vi "GT Buf Event Off.vi"(6 "fifo":i16, 7 "count":i16, 8 "error in (no error)":errorcluster caption="错误输入（无错误）", 9 "eventIndex":i16, 10 "crd":i16, 11 "cardNum":i16) -> (0 "error out":errorcluster caption="错误输出", 3 "function return":i16)   [LabVIEW 2020, in "gts1.lvlib"]
doc: "GT_API GT_BufEventOff(short cardNum,short crd,short eventIndex,short count,short fifo);"
uses:
  gts1.lvlib
  dll/32bit/multi_card/gts.dll
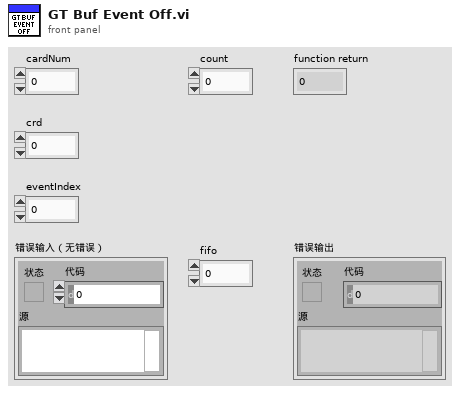
[diagram p1: front panel]
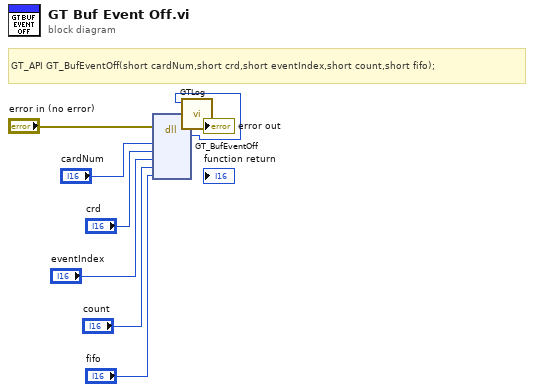
[diagram p0: block diagram]
diagram:
  # "GT_API GT_BufEventOff(short cardNum,short crd,short eventIndex,short count,short fifo);"
  n1 = dll-call lib="D:/Git/GoogolCard/dll/32bit/multi_card/gts.dll" fn="GT_BufEventOff"(error in="error in (no error)", "cardNum"="cardNum", "crd"="crd", "eventIndex"="eventIndex", "count"="count", "fifo"="fifo") -> (error out=w3:errorcluster, w1:i16)  [unwired: 7 in, 1 out]
  n2 = call "GTLog.vi"("error in (no error)"=w3, "Numeric"=w1) -> ("error out"=→"error out":errorcluster)  [unwired: 9 in]
